vi "LED Matrix Display.vi"(4 "Brightness":u8=50 max=100 step=1, 6 "Factor":dbl=2.5, 8 "error in":errorcluster, 10 "image depth":i32, 11 "image":u8[](array[numeric])) -> (0 "error out":errorcluster, 5 "LED Matrix":picture)   [LabVIEW 2013]
uses:
  <vilib>/FPGAPlugInAG/myRIO-1900/niLvFpga_Open_myRIO-1900.vi
  <vilib>/rvi/interface/common/dynamic/niFpgaDynamicAddResources.vi
  <vilib>/myRIO/Common/Instrument Driver Framework/Utilities/vis/FPGA Ref Manager.vi
  <vilib>/Utility/error.llb/Error Cluster From Error Code.vi
  <vilib>/FPGAPlugInAG/Dynamic/niLvFpga_Close_Dynamic.vi
  <vilib>/rvi/interface/nirviOpenFPGA/nirviOpenFPGA.xnode
  FPGA Bitfiles/LEDMatrix4_FPGATarget_myRIO-1900Custom_r1aLzQW2H5E.lvbitx
  <vilib>/rvi/interface/nirviCloseFPGA/nirviCloseFPGA.xnode
  <vilib>/myRIO/Instrument Drivers/Utilities/Utilities.lvlib
panel:
  # "Image Data"
  # "Image Depth: Only 24 bit and 32 bit\nis currently supported. For 32 bit, the\nlow byte is alpha and thrown away."
  # "Adjusts Brightness/Contrast with a\nlogarithmic scale to better match \nperception. Number is a floating point\nand smaller numbers, like 2.5 may work best.\nSet to 1 to be unity and disable the effect."
  # "Brightness Level from 0 (off) to 100 (max).\nToo bright may cause robot batteries to\ndischarge too quickly and too dim may lose\ncolors."
  # "Optional output. This shows the image\nthat should be displayed on the LED Matrix."
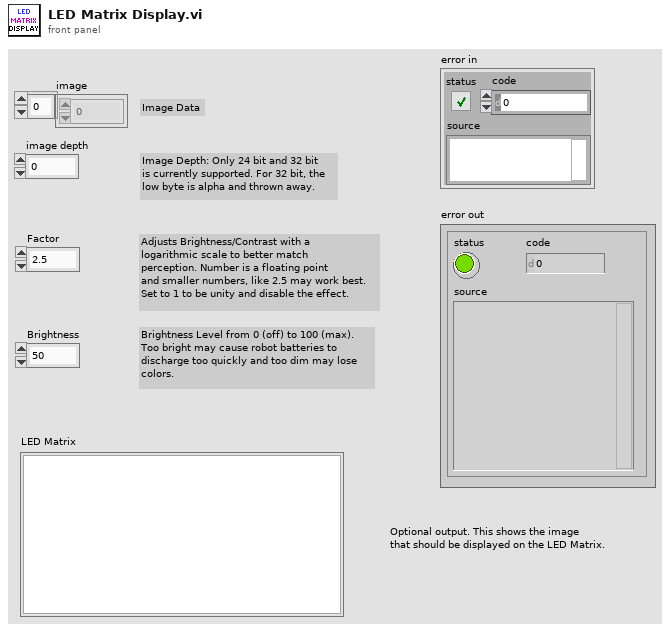
[diagram p1: front panel]
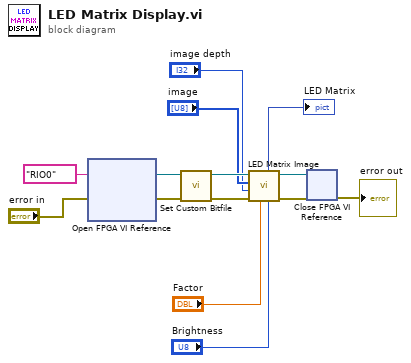
[diagram p0: block diagram]
diagram:
  n1 = xnode "Open FPGA VI Reference"("error in"="error in", "resource name"=tag "RIO0") -> ("FPGA VI Reference Out"=w13:refnum<k20>, "error out"=w14:errorcluster)
  n2 = call <vilib>:"Set Custom Bitfile.vi"("error in (no error)"=w14, "Customized FPGA Reference in"=w13) -> ("error out"=w9:errorcluster, "Customized FPGA Reference out"=w10:refnum<k20>)  [unwired: 8 in]
  n3 = call "LED Matrix Image.vi"("Brightness"="Brightness", "Factor"="Factor", "error in (no error)"=w9, "image depth"="image depth", "image"="image", "Refnum in"=w10) -> ("error out"=w6:errorcluster, "Refnum out"=w4:refnum<k20>, "LED Matrix"=→"LED Matrix":picture)  [unwired: 3 in]
  n4 = xnode "Close FPGA VI Reference"("FPGA VI Reference In"=w4, "error in"=w6) -> ("error out"=→"error out":errorcluster)
